vi "Read Diagnostic Configuration (XML).vi"(8 "error in (no error)":errorcluster, 11 "Path in":path) -> (0 "error out":errorcluster, 3 "Configuration":T1 {"DID Outputs"."Frames"."Signals"."Byte Order" items=["Little Endian", "Big Endian"]; "DID Outputs"."Frames"."Signals"."Data Type" items=["Signed", "Unsigned", "IEEE Float"]; "Memory Inputs"."Frames"."Signals"."Byte Order" items=["Little Endian", "Big Endian"]; "Memory Inputs"."Frames"."Signals"."Data Type" items=["Signed", "Unsigned", "IEEE Float"]; "Memory Outputs"."Frames"."Signals"."Byte Order" items=["Little Endian", "Big Endian"]; "Memory Outputs"."Frames"."Signals"."Data Type" items=["Signed", "Unsigned", "IEEE Float"]; "Routines"."Routine Array"."Stop Parameters"."Response"."Byte Order" items=["Little Endian", "Big Endian"]; "Routines"."Routine Array"."Stop Parameters"."Response"."Data Type" items=["Signed", "Unsigned", "IEEE Float"]; "Routines"."Routine Array"."Stop Parameters"."Cmd"."Byte Order" items=["Little Endian", "Big Endian"]; "Routines"."Routine Array"."Stop Parameters"."Cmd"."Data Type" items=["Signed", "Unsigned", "IEEE Float"]; "Routines"."Routine Array"."Request Parameters"."Response"."Byte Order" items=["Little Endian", "Big Endian"]; "Routines"."Routine Array"."Request Parameters"."Response"."Data Type" items=["Signed", "Unsigned", "IEEE Float"]; "Routines"."Routine Array"."Request Parameters"."Cmd"."Byte Order" items=["Little Endian", "Big Endian"]; "Routines"."Routine Array"."Request Parameters"."Cmd"."Data Type" items=["Signed", "Unsigned", "IEEE Float"]; "Routines"."Routine Array"."Start Parameters"."Response"."Byte Order" items=["Little Endian", "Big Endian"]; "Routines"."Routine Array"."Start Parameters"."Response"."Data Type" items=["Signed", "Unsigned", "IEEE Float"]; "Routines"."Routine Array"."Start Parameters"."Cmd"."Byte Order" items=["Little Endian", "Big Endian"]; "Routines"."Routine Array"."Start Parameters"."Cmd"."Data Type" items=["Signed", "Unsigned", "IEEE Float"]; "IO Controls"."IO Control Array"."Signals"."Response"."Byte Order" items=["Little Endian", "Big Endian"]; "IO Controls"."IO Control Array"."Signals"."Response"."Data Type" items=["Signed", "Unsigned", "IEEE Float"]; "IO Controls"."IO Control Array"."Signals"."Cmd"."Byte Order" items=["Little Endian", "Big Endian"]; "IO Controls"."IO Control Array"."Signals"."Cmd"."Data Type" items=["Signed", "Unsigned", "IEEE Float"]; "DTC"."DTC Control"."Signals"."Byte Order" items=["Little Endian", "Big Endian"]; "DTC"."DTC Control"."Signals"."Data Type" items=["Signed", "Unsigned", "IEEE Float"]; "Diagnostics Basic Configuraiton"."IO Mode" items=["CAN 2.0", "CAN FD", "CAN FD+BRS"]; "Diagnostics Basic Configuraiton"."Fill Byte" format="%.0x"; "Diagnostics Basic Configuraiton"."VW TP Channel ID" format="%.0x"; "Diagnostics Basic Configuraiton"."Receive UUDT ID" format="%.0x"; "Diagnostics Basic Configuraiton"."Receive Extension" format="%.0x"; "Diagnostics Basic Configuraiton"."Transmit Extension" format="%.0x"; "Diagnostics Basic Configuraiton"."Receive ID" format="%.0x"; "Diagnostics Basic Configuraiton"."Transmit ID" format="%.0x"; "DID Inputs"."Frames"."Signals"."Byte Order" items=["Little Endian", "Big Endian"]; "DID Inputs"."Frames"."Signals"."Data Type" items=["Signed", "Unsigned", "IEEE Float"]; "PID Inputs"."Frames"."Signals"."Byte Order" items=["Little Endian", "Big Endian"]; "PID Inputs"."Frames"."Signals"."Data Type" items=["Signed", "Unsigned", "IEEE Float"]; "PID Outputs"."Frames"."Signals"."Byte Order" items=["Little Endian", "Big Endian"]; "PID Outputs"."Frames"."Signals"."Data Type" items=["Signed", "Unsigned", "IEEE Float"]})   [LabVIEW 2019, in "Diagnostics Addon SysDef API.lvlib"]
uses:
  Diagnostics Addon SysDef API.lvlib
  System Explorer/Types/SysDef.Export.ctl
  Shared/Types/CAN.ctl
  Shared/Types/CAN.Interface.ctl
  Shared/Types/Protocol.ctl
  Shared/Types/Transport.ctl
  Shared/Types/Security.ctl
  System Explorer/Types/Frames.Export.ctl
  System Explorer/Types/Frame.Export.ctl
  Shared/Types/Signal.ctl
  System Explorer/Types/DPIDs.Export.ctl
  System Explorer/Types/DPID.Export.ctl
  Shared/Types/DPID.ctl
  Shared/Types/DPID.Rate.ctl
  System Explorer/Types/DTC.Export.ctl
  Shared/Types/DTC.Settings.ctl
  Shared/Types/DTC.Descriptor.ctl
  System Explorer/Types/DTCControl.Export.ctl
  Shared/Types/986x.ctl
  System Explorer/Types/Command.Export.ctl
  System Explorer/Types/Status.Export.ctl
  System Explorer/Types/IOControls.Export.ctl
  System Explorer/Types/IO.Export.ctl
  System Explorer/Types/CmdResp.Export.ctl
  System Explorer/Types/Routines.Export.ctl
  System Explorer/Types/Routine.Export.ctl
  System Explorer/Types/UserDefined.Export.ctl
  System Explorer/Types/UserDefined.Group.Export.ctl
  System Explorer/Types/UserDefined.Group.Message.Export.ctl
  System Explorer/Diagnostics Addon System Explorer.lvlib
  Shared/Diagnostics Addon Shared.lvlib
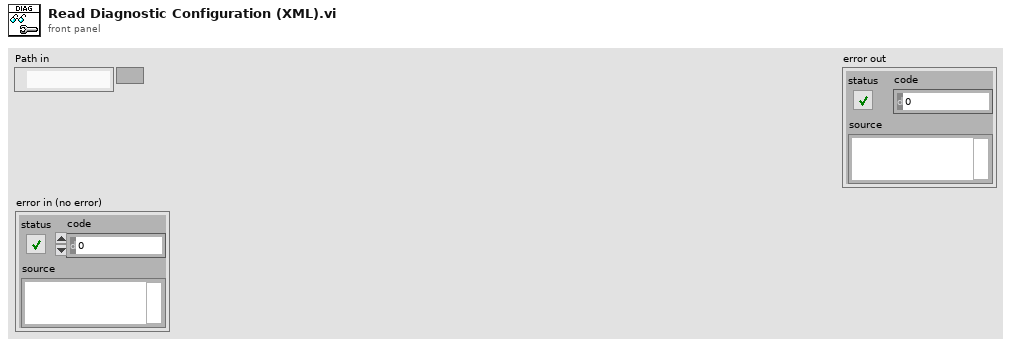
[diagram p1: front panel]
types:
  T1 = typedef "Diagnostics Addon System Explorer.lvlib/SysDef.Export.ctl" = cluster{"Name":string, "Description":string, "Diagnostics Basic Configuraiton":T2, "DID Outputs":T7, "DID Inputs":T7, "PID Outputs":T7, "PID Inputs":T7, "DPIDs":T10, "DTC":T14, "NI 986x Support":T18, "Commands":T19, "Status":T20, "IO Controls":T21, "Routines":T24, "Memory Outputs":T7, "Memory Inputs":T7, "User Defined":T26}
  T2 = typedef "Diagnostics Addon Shared.lvlib/CAN.ctl" = cluster{"Interface":T3, "Baud Rate":u64, "Diagnostic Protocol":T4, "Transport Protocol":T5, "Transmit ID":u32, "Receive ID":u32, "Transmit Extension":u8, "Receive Extension":u8, "Receive UUDT ID":u32, "Enable Stream":bool, "VW TP Channel ID":u32, "Fill Frame":bool, "Fill Byte":u8, "Termination":bool, "LIN Cluster":refnum<k21>, "NAD":u8, "IO Mode":u32, "Max DLC":u16, "FD Baud Rate":u64, "Security":T6}
  T3 = typedef "Diagnostics Addon Shared.lvlib/CAN.Interface.ctl" = string
  T4 = typedef "Diagnostics Addon Shared.lvlib/Protocol.ctl" = enum16{"GMLAN", "KWP-2000", "UDS", "User-Defined"}
  T5 = typedef "Diagnostics Addon Shared.lvlib/Transport.ctl" = enum16{"ISO TP - Normal Mode", "ISO TP - Mixed Mode", "VW TP 2.0", "Diagnostics on IP", "ISO TP LIN"}
  T6 = typedef "Diagnostics Addon Shared.lvlib/Security.ctl" = cluster{"Source DLL Path":path, "Security Level":u8, "Target DLL Path":path}
  T7 = typedef "Diagnostics Addon System Explorer.lvlib/Frames.Export.ctl" = cluster{"Description":string, "Frames":T8[]}
  T8 = typedef "Diagnostics Addon System Explorer.lvlib/Frame.Export.ctl" = cluster{"Name":string, "Description":string, "ID":u32, "Signals":T9[]}
  T9 = typedef "Diagnostics Addon Shared.lvlib/Signal.ctl" = cluster{"Start Bit":u32, "Length":u32, "Scaling Factor":dbl, "Scaling Offset":dbl, "Minimum":dbl, "Maximum":dbl, "Data Type":u32, "Byte Order":u32, "Default Value":dbl, "Name":string, "Units":string, "Description":string}
  T10 = typedef "Diagnostics Addon System Explorer.lvlib/DPIDs.Export.ctl" = cluster{"Description":string, "DPIDs":T11[]}
  T11 = typedef "Diagnostics Addon System Explorer.lvlib/DPID.Export.ctl" = cluster{"Name":string, "Description":string, "DPID":T12}
  T12 = typedef "Diagnostics Addon Shared.lvlib/DPID.ctl" = cluster{"DPID ID":u8, "Speed":T13, "PIDs":u16[]}
  T13 = typedef "Diagnostics Addon Shared.lvlib/DPID.Rate.ctl" = enum16{"Slow", "Medium", "Fast"}
  T14 = typedef "Diagnostics Addon System Explorer.lvlib/DTC.Export.ctl" = cluster{"Description":string, "Settings":T15, "DTC Control":T17, "Created DTCs":u32}
  T15 = typedef "Diagnostics Addon Shared.lvlib/DTC.Settings.ctl" = cluster{"Descriptor":T16, "Value.Code":dbl[], "Value.String":string[], "Value.J2012String":string[], "Status.Code":dbl[], "Status.String":string[]}
  T16 = typedef "Diagnostics Addon Shared.lvlib/DTC.Descriptor.ctl" = cluster{"DTC Byte Length":i32, "Status Byte Length":i32, "Add Data Byte Length":i32, "Byte Order":enum16{"Motorola", "Intel"}}
  T17 = typedef "Diagnostics Addon System Explorer.lvlib/DTCControl.Export.ctl" = cluster{"Description":string, "Signals":T9[]}
  T18 = typedef "Diagnostics Addon Shared.lvlib/986x.ctl" = cluster{"Enable":bool, "RIO Device":string, "Bitfile":path}
  T19 = typedef "Diagnostics Addon System Explorer.lvlib/Command.Export.ctl" = cluster{"Description":string}
  T20 = typedef "Diagnostics Addon System Explorer.lvlib/Status.Export.ctl" = cluster{"Description":string}
  T21 = typedef "Diagnostics Addon System Explorer.lvlib/IOControls.Export.ctl" = cluster{"Description":string, "IO Control Array":T22[]}
  T22 = typedef "Diagnostics Addon System Explorer.lvlib/IO.Export.ctl" = cluster{"Name":string, "Description":string, "ID":u16, "Signals":T23}
  T23 = typedef "Diagnostics Addon System Explorer.lvlib/CmdResp.Export.ctl" = cluster{"Cmd":T9[], "Response":T9[]}
  T24 = typedef "Diagnostics Addon System Explorer.lvlib/Routines.Export.ctl" = cluster{"Description":string, "Routine Array":T25[]}
  T25 = typedef "Diagnostics Addon System Explorer.lvlib/Routine.Export.ctl" = cluster{"Name":string, "Description":string, "ID":u16, "Start Parameters":T23, "Request Parameters":T23, "Stop Parameters":T23}
  T26 = typedef "Diagnostics Addon System Explorer.lvlib/UserDefined.Export.ctl" = cluster{"Description":string, "Groups":T27[]}
  T27 = typedef "Diagnostics Addon System Explorer.lvlib/UserDefined.Group.Export.ctl" = cluster{"Name":string, "Description":string, "Messages":T28[]}
  T28 = typedef "Diagnostics Addon System Explorer.lvlib/UserDefined.Group.Message.Export.ctl" = cluster{"Name":string, "Description":string, "Signals":T23}
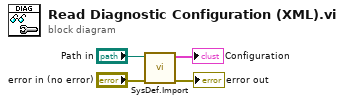
[diagram p0: block diagram]
diagram:
  n1 = call "SysDef.Import.vi"("error in (no error)"="error in (no error)", "Path in"="Path in") -> ("error out"=→"error out":errorcluster, "Configuration"=→"Configuration":T1)  [unwired: 8 in]
